vi "rqcAlice Attenuator Stress Test (Host).vi"() -> ()   [LabVIEW 2018]
uses:
  <vilib>/FPGAPlugInAG/PCIe-7820R/niLvFpga_Open_PCIe-7820R.vi
  <vilib>/rvi/interface/common/dynamic/niFpgaDynamicAddResources.vi
  <vilib>/FPGAPlugInAG/Dynamic/niLvFpga_Close_Dynamic.vi
  <vilib>/rvi/interface/nirviOpenFPGA/nirviOpenFPGA.xnode
  FPGA Bitfiles/rqcAlice FPGA (7820R) v 2.3.0.lvbitx
  <vilib>/rvi/interface/nirviCloseFPGA/nirviCloseFPGA.xnode
  Automated Measurements/KeySight 8164B LAN InstrLib.lvlib
panel:
  in  "Step period, mS":u32=500
  out "Att Requested, dB":fxp<+,7,6>
  in  "delta step, dB":fxp<+,7,6>=5.0
  out "Att Measured, dB":dbl
  out "Base Power, dBm":dbl
  out "Hung":bool
  out "Att Delta":dbl(graph)
  in  "acceptable Att difference":dbl=2.0
  out "error out":errorcluster
  in  "stop":bool
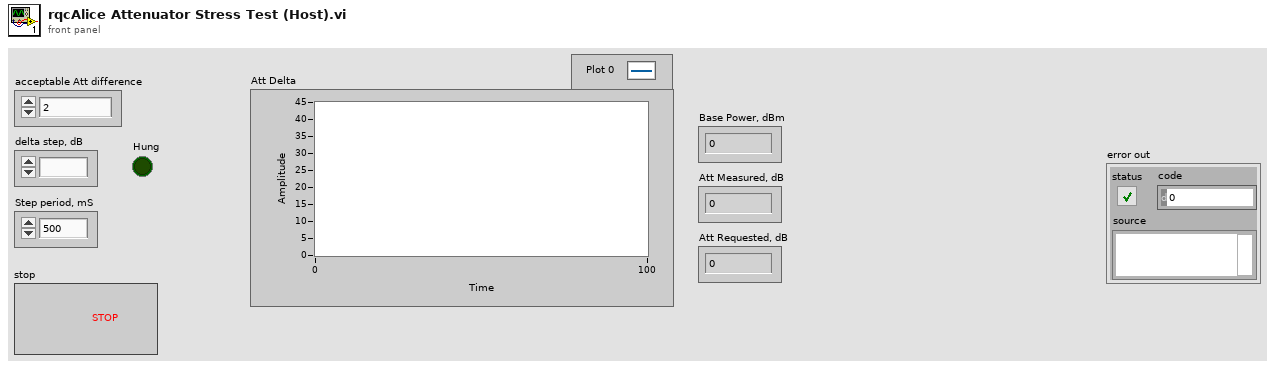
[diagram p1: front panel]
types:
  T1 = typedef "KeySight 8164B LAN InstrLib.lvlib/KeySight 8164B control.ctl" = cluster{"Connection ID":refnum<k5>, "Connected":bool, "Info":string, "Slots Info":string[]}
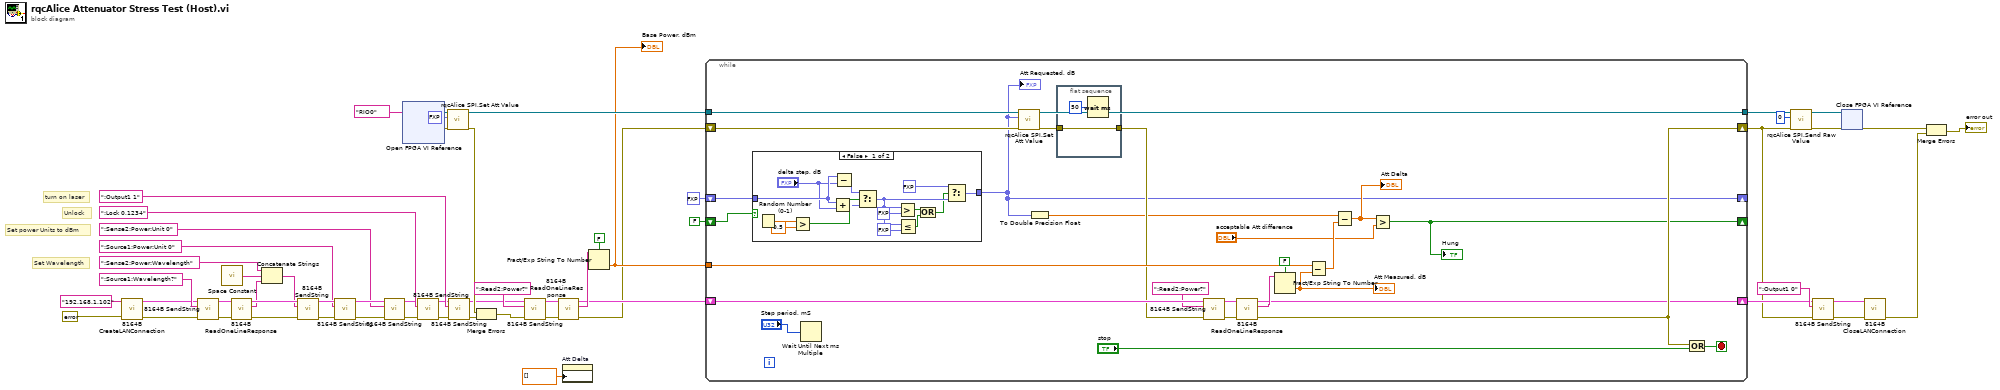
[diagram p0: block diagram]
diagram:
  # "Unlock"
  # "turn on laser"
  # "Set power Units to dBm"
  # "Set Wavelength"
  n1 = call "8164B CreateLANConnection.vi"("error in"=errorcluster {"status"=FALSE, "code"=0, "source"=""}, "IP address"="192.168.1.102" ("address")) -> ("error out"=w35:errorcluster, "KeySight 8164B control out"=w34:T1)  [unwired: 8 in]
  n2 = call "8164B SendString.vi"("error in"=w35, "CMD"=":Source1:Wavelength?", "KeySight 8164B control in"=w34) -> ("error out"=w49:errorcluster, "KeySight 8164B control out"=w50:T1)  [unwired: 7 in]
  n3 = call <vilib>:"Space Constant.vi"() -> ("String"=w44:string)
  n4 = call "8164B ReadOneLineResponse.vi"("error in"=w49, "KeySight 8164B control in"=w50) -> ("error out"=w46:errorcluster, "OneLineResponse"=w43:string, "KeySight 8164B control out"=w47:T1)  [unwired: 7 in]
  n5 = Concatenate Strings(":Sense2:Power:Wavelength" ("CMD"), w44, w43) -> (w42:string)
  n6 = call "8164B SendString.vi"("error in"=w46, "CMD"=w42, "KeySight 8164B control in"=w47) -> ("error out"=w40:errorcluster, "KeySight 8164B control out"=w41:T1)  [unwired: 7 in]
  n7 = call "8164B SendString.vi"("error in"=w40, "CMD"=":Source1:Power:Unit 0", "KeySight 8164B control in"=w41) -> ("error out"=w37:errorcluster, "KeySight 8164B control out"=w38:T1)  [unwired: 7 in]
  n8 = call "8164B SendString.vi"("error in"=w37, "CMD"=":Sense2:Power:Unit 0", "KeySight 8164B control in"=w38) -> ("error out"=w5:errorcluster, "KeySight 8164B control out"=w7:T1)  [unwired: 7 in]
  n9 = xnode "Open FPGA VI Reference"("resource name"=tag "RIO0") -> ("FPGA VI Reference Out"=w33:refnum<k20>, "error out"=w31:errorcluster)  [unwired: 1 in]
  n10 = call "8164B SendString.vi"("error in"=w5, "CMD"=":Lock 0,1234", "KeySight 8164B control in"=w7) -> ("error out"=w4:errorcluster, "KeySight 8164B control out"=w6:T1)  [unwired: 7 in]
  n11 = call "rqcAlice SPI.Set Att Value.vi"("error in"=w31, "Attenuation, dB"=fxp<+,7,6> 0.0, "Alice FPGA Reference In"=w33) -> ("error out"=w22:errorcluster, "Alice FPGA Reference Out"=w32:refnum<k20>)  [unwired: 7 in]
  n12 = call "8164B SendString.vi"("error in"=w4, "CMD"=":Output1 1", "KeySight 8164B control in"=w6) -> ("error out"=w20:errorcluster, "KeySight 8164B control out"=w19:T1)  [unwired: 7 in]
  n13 = Merge Errors(w22, w20) -> (w23:errorcluster)
  n14 = call "8164B SendString.vi"("error in"=w23, "CMD"=":Read2:Power?", "KeySight 8164B control in"=w19) -> ("error out"=w30:errorcluster, "KeySight 8164B control out"=w28:T1)  [unwired: 7 in]
  n15 = call "8164B ReadOneLineResponse.vi"("error in"=w30, "KeySight 8164B control in"=w28) -> ("error out"=w21:errorcluster, "OneLineResponse"=w27:string, "KeySight 8164B control out"=w24:T1)  [unwired: 7 in]
  n16 = property on="Att Delta" class="WFChart (strict)"("History Data"=dbl[] []) -> ()  [unwired: 2 in, 2 out]
  n17 = Fract/Exp String To Number(use system decimal point (T)=FALSE, string=w27) -> (number=w25:dbl)  [unwired: 2 in, 1 out]
  "Base Power, dBm" <- w25
  n18 = while {
    tunnel: w32 -> [w71]
    shift-right: [w80] -> w14
    shift-left: w21 -> [w69]
    tunnel: [w70] -> w53
    tunnel: w25 -> [w79]
    shift-right: [w67] -> w16
    shift-left: w24 -> [w82]
    shift-right: [w60] -> _
    shift-left: fxp<+,7,6> 20.0 ("t") -> [w62]
    shift-right: [w59] -> _
    shift-left: FALSE -> [w58]
    stop <- w83 stop-if-true
    n19 = case shown="False" w58 {
      tunnel: w62 -> [w96 w99]
      tunnel: [w90 w99] -> w60
      frame False {
        n20 = Random Number (0-1)() -> (number: 0 to 1=w98:dbl)
        n21 = Greater?(x=w98, y=0.5) -> (0:w94:bool)
        n22 = Add(x=w96, y="delta step, dB") -> (x+y=w93:fxp<+,7,6>)
        n23 = Subtract(x=w96, y="delta step, dB") -> (x-y=w92:fxp<+,7,6>)
        n24 = Select(t=w92, s=w94, f=w93) -> (s? t:f=w87:fxp<+,7,6>)
        n25 = Greater?(x=w87, y=fxp<+,7,6> 40.0) -> (0:w88:bool)
        n26 = Less Or Equal?(x=w87, y=fxp<+,7,6> 0.0) -> (x <= y?=w84:bool)
        n27 = Compound Arithmetic op=OR(w88, w84) -> (w85:bool)
        n28 = Select(t=fxp<+,7,6> 20.0, s=w85, f=w87) -> (s? t:f=w90:fxp<+,7,6>)
      }
      frame True {
      }
    }
    "Att Requested, dB" <- w60
    n29 = Wait Until Next ms Multiple(millisecond multiple="Step period, mS") -> ()  [unwired: 1 out]
    n30 = call "rqcAlice SPI.Set Att Value.vi"("error in"=w69, "Attenuation, dB"=w60, "Alice FPGA Reference In"=w71) -> ("error out"=w68:errorcluster, "Alice FPGA Reference Out"=w70:refnum<k20>)  [unwired: 7 in]
    n31 = To Double Precision Float(number=w60) -> (double precision float=w61:dbl)
    n32 = flat-sequence {
      tunnel: w68 -> [w101]
      tunnel: [w101] -> w78
      frame #0 {
        n33 = Wait (ms)(milliseconds to wait=u32 50) -> ()  [unwired: 1 out]
      }
    }
    n34 = call "8164B SendString.vi"("error in"=w78, "CMD"=":Read2:Power?", "KeySight 8164B control in"=w82) -> ("error out"=w75:errorcluster, "KeySight 8164B control out"=w77:T1)  [unwired: 7 in]
    n35 = call "8164B ReadOneLineResponse.vi"("error in"=w75, "KeySight 8164B control in"=w77) -> ("error out"=w80:errorcluster, "OneLineResponse"=w73:string, "KeySight 8164B control out"=w67:T1)  [unwired: 7 in]
    n36 = Fract/Exp String To Number(use system decimal point (T)=FALSE, string=w73) -> (number=w72:dbl)  [unwired: 2 in, 1 out]
    "Att Measured, dB" <- w72
    n37 = Subtract(x=w79, y=w72) -> (x-y=w66:dbl)
    n38 = Subtract(x=w61, y=w66) -> (x-y=w65:dbl)
    "Att Delta" <- w65
    n39 = Greater?(x=w65, y="acceptable Att difference") -> (0:w59:bool)
    "Hung" <- w59
    n40 = Compound Arithmetic op=OR(w80, "stop") -> (w83:bool)
  }
  n41 = call "rqcAlice SPI.Send Raw Value.vi"("error in"=w14, "value"=u16 0, "Alice FPGA Reference In"=w53) -> ("error out"=w13:errorcluster, "Alice FPGA Reference Out"=w52:refnum<k20>)  [unwired: 7 in]
  n42 = call "8164B SendString.vi"("error in"=w14, "CMD"=":Output1 0", "KeySight 8164B control in"=w16) -> ("error out"=w15:errorcluster, "KeySight 8164B control out"=w12:T1)  [unwired: 7 in]
  n43 = xnode "Close FPGA VI Reference"("FPGA VI Reference In"=w52, "error in"=w13) -> ("error out"=w56:errorcluster)
  n44 = call "8164B CloseLANConnection.vi"("error in"=w15, "KeySight 8164B control"=w12) -> ("error out"=w10:errorcluster)  [unwired: 9 in]
  n45 = Merge Errors(w56, w10) -> (→"error out":errorcluster)
